vi "Server.vi"() -> ()   [LabVIEW 2020]
uses:
  Queue Type.ctl
panel:
  in  "Send this value:":T1
  in  "stop":bool
  # "Start Client.vi running first, then run this VI."
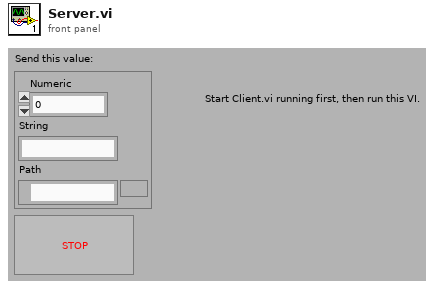
[diagram p1: front panel]
types:
  T1 = typedef "Queue Type.ctl" = cluster{"Numeric":dbl, "String":string, "Path":path}
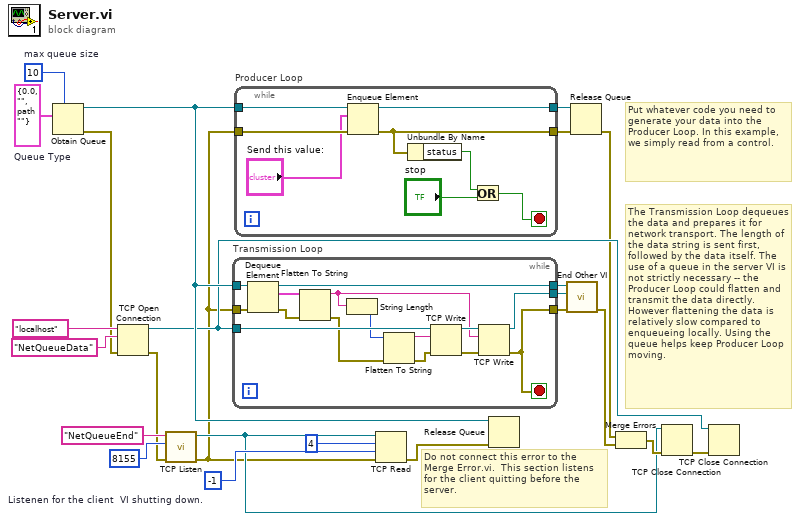
[diagram p0: block diagram]
diagram:
  w1 = 10  # max queue size
  w18 = -1  # Listenen for the client  VI shutting down.
  w23 = T1 {"Numeric"=0.0, "String"="", "Path"=path ""}  # Queue Type
  # "The Transmission Loop dequeues the data and prepares it for network transport. The length of the data string is sent first, followed by the data itself. The use of a queue in the server VI is not strictly necessary -- the Producer Loop could flatten and transmit the data directly. However flattening the data is relatively slow compared to enqueueing locally. Using the queue helps keep Producer Loop moving."
  # "Put whatever code you need to generate your data into the Producer Loop. In this example, we simply read from a control."
  # "Do not connect this error to the Merge Error.vi.  This section listens for the client quitting before the server."
  n1 = Obtain Queue(max queue size (-1, unlimited)=w1, element data type=w23) -> (queue out=w16:refnum<queue>, error out=w7:errorcluster)  [unwired: 2 in, 2 out]
  n2 = TCP Open Connection(address="localhost", remote port or service name="NetQueueData" ("address"), error in (no error)=w7) -> (connection ID=w11:refnum<k5>, error out=w6:errorcluster)  [unwired: 2 out]
  n3 = call <vilib>:"TCP Listen.vi"("error in (no error)"=w6, "port"=u16 8155, "service name"="NetQueueEnd" ("address")) -> ("error out"=w5:errorcluster, "connection ID"=w13:refnum<k5>)  [unwired: 1 in, 6 out]
  n4 = while "Transmission Loop" {
    tunnel: w16 -> [w39]
    tunnel: w11 -> [w32]
    tunnel: w5 -> [w38]
    tunnel: [w35] -> w21
    tunnel: [w34] -> w22
    tunnel: [w33] -> w20
    stop <- w34 stop-if-true
    n5 = Dequeue Element(queue=w39, error in (no error)=w38) -> (queue out=w35:refnum<queue>, element=w36:T1, error out=w37:errorcluster)  [unwired: 2 out]
    n6 = Flatten To String(anything=w36, error in (no error)=w37) -> (data string=w29:string, error out=w25:errorcluster)  [unwired: 3 out]
    n7 = String Length(string=w29) -> (length=w28:i32)
    n8 = Flatten To String(anything=w28, error in (no error)=w25) -> (data string=w27:string, error out=w26:errorcluster)  [unwired: 3 out]
    n9 = TCP Write(connection ID=w32, data in=w27, error in (no error)=w26) -> (connection ID out=w31:refnum<k5>, error out=w30:errorcluster)  [unwired: 2 out]
    n10 = TCP Write(connection ID=w31, data in=w29, error in (no error)=w30) -> (connection ID out=w33:refnum<k5>, error out=w34:errorcluster)  [unwired: 2 out]
  }
  n11 = while "Producer Loop" {
    tunnel: w16 -> [w47]
    tunnel: w5 -> [w46]
    tunnel: [w45] -> w4
    tunnel: [w42] -> w2
    stop <- w44 stop-if-true
    n12 = Enqueue Element(queue=w47, element="Send this value:", error in (no error)=w46) -> (queue out=w45:refnum<queue>, error out=w42:errorcluster)  [unwired: 2 out]
    n13 = Unbundle By Name(w42) -> ("status"=w41:bool)
    n14 = Or(x=w41, y="stop") -> (x .or. y?=w44:bool)
  }
  n15 = TCP Read(connection ID=w13, bytes to read=4, error in (no error)=w5, 9:w18) -> (error out=w17:errorcluster)  [unwired: 3 out]
  n16 = Release Queue(queue=w16, error in (no error)=w17) -> ()  [unwired: 4 out]
  n17 = call "End Other VI.vi"("error in (no error)"=w22, "TCP Connection"=w20, "queue in"=w21) -> ("error out"=w15:errorcluster)  [unwired: 8 out]
  n18 = Release Queue(queue=w4, error in (no error)=w2) -> (error out=w3:errorcluster)  [unwired: 3 out]
  n19 = Merge Errors(w3, w15) -> (w14:errorcluster)
  n20 = TCP Close Connection(connection ID=w13, error in (no error)=w14) -> (error out=w12:errorcluster)  [unwired: 2 out]
  n21 = TCP Close Connection(connection ID=w11, error in (no error)=w12) -> ()  [unwired: 3 out]
